vi "fromString.vi"(9 "DateTime String":string, 11 "DateTimeFormatter in":refnum<class "DateTimeFormatter.lvclass">) -> (1 "Timestamp":timestamp, 3 "DateTimeFormatter out":refnum<class "DateTimeFormatter.lvclass">)   [LabVIEW 2018, in "DateTimeFormatter.lvclass"]
uses:
  DateTimeFormatter.lvclass
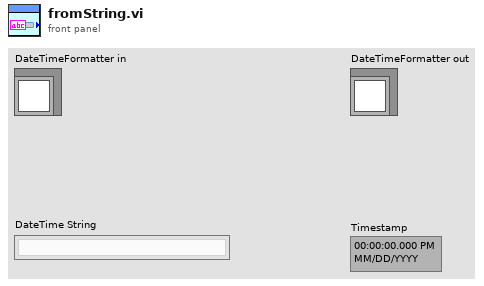
[diagram p1: front panel]
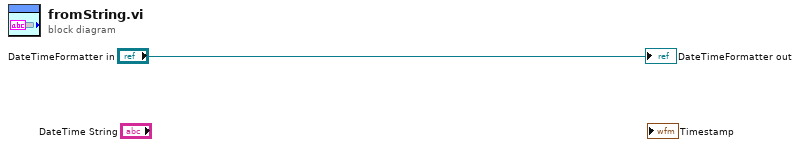
[diagram p0: block diagram]
diagram:
  "DateTimeFormatter out" <- "DateTimeFormatter in"
